vi "Request Supported.vi"(8 "error in (no error)":errorcluster, 10 "Request":refnum<class "Request.lvclass">, 11 "SOL Auth in":refnum<class "SOL Auth.lvclass">) -> (0 "error out":errorcluster, 2 "Supported":bool, 3 "SOL Auth out":refnum<class "SOL Auth.lvclass">)   [LabVIEW 2020, in "Summer of LabVIEW.lvlib" / "SOL Auth.lvclass"]
uses:
  SOL Auth.lvclass
  <vilib>/IlluminatedG/IG HTTP Utils/HTTP Utils/Request/Request.lvclass
  <vilib>/IlluminatedG/IG HTTP Utils/HTTP Utils/Method.ctl
  SOL Auth.lvclass/SOL Auth.ctl
  <vilib>/IlluminatedG/lv-stream/URI/URI.lvclass
  <vilib>/IlluminatedG/IG HTTP Utils/HTTP Utils/HTTP Utils.lvlib
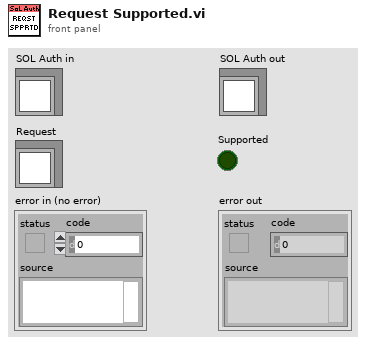
[diagram p1: front panel]
types:
  T1 = typedef "HTTP Utils.lvlib/Method.ctl" = enum16{"GET", "HEAD", "POST", "PUT", "DELETE", "CONNECT", "OPTIONS", "TRACE", "PATCH"}
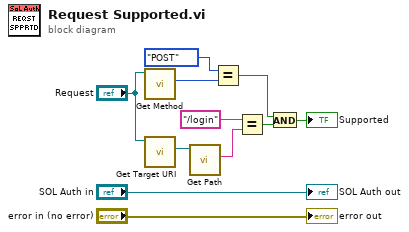
[diagram p0: block diagram]
diagram:
  n1 = call <vilib>:"Get Method.vi"("Request in"="Request") -> ("Method"=w5:T1)  [unwired: 8 in, 2 out]
  n2 = call <vilib>:"Get Target URI.vi"("Request in"="Request") -> ("Target URI"=w9:refnum<class "URI.lvclass">)  [unwired: 8 in, 2 out]
  n3 = call <vilib>:"Get Path.vi"("URI in"=w9) -> ("Path"=w8:string)  [unwired: 8 in, 2 out]
  n4 = Equal?(x=Method."POST", y=w5) -> (x = y?=w2:bool)
  n5 = Equal?(x="/login", y=w8) -> (x = y?=w3:bool)
  n6 = And(x=w2, y=w3) -> (x .and. y?=→"Supported":bool)
  "error out" <- "error in (no error)"
  "SOL Auth out" <- "SOL Auth in"
